vi "_Update LDAC.vi"   [LabVIEW 2012]
uses:
  <vilib>/eio/EIONode/EIONode.xnode
  Instance           1 20Saved   _Update LDAC .vi
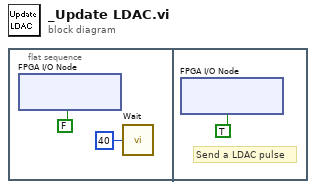
[diagram p0: block diagram]
diagram:
  n1 = flat-sequence {
    frame #0 {
      n2 = xnode "FPGA I/O Node"("Port7/DIO2"=FALSE ("Digital Out")) -> ()  [unwired: 1 in, 1 out]
      n3 = call "Wait"("Count(Ticks)"=u8 40) -> ()  [unwired: 1 out]
    }
    frame #1 {
      # "Send a LDAC pulse"
      n4 = xnode "FPGA I/O Node"("Port7/DIO2"=TRUE ("Digital Out")) -> ()  [unwired: 1 in, 1 out]
    }
  }
